vi "Unregister.vi"(8 "Error In":errorcluster, 10 "Registrant Enq":refnum<class "Message Enqueuer.lvclass">, 11 "Event Source In":refnum<class "Event Source Actor.lvclass">) -> (0 "Error Out":errorcluster, 3 "Event Source Out":refnum<class "Event Source Actor.lvclass">)   [LabVIEW 2021, in "EventSourceActor.lvlib" / "Event Source.lvlib" / "Event Source Actor.lvclass"]
doc: "This method unregisters a specific Actors Enqueuer from all Events he is listening to from this Event Source Actor."
uses:
  Event Source Actor.lvclass
  <vilib>/ActorFramework/Message Enqueuer/Message Enqueuer.lvclass
  Event Source Actor.lvclass/Event Source Actor.ctl
  48172011-38dd-4e95-b88c-c50fd512a03c.vi
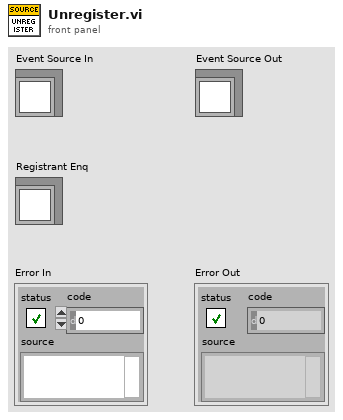
[diagram p1: front panel]
types:
  T1 = map{string, set{refnum<class "Message Enqueuer.lvclass">}}
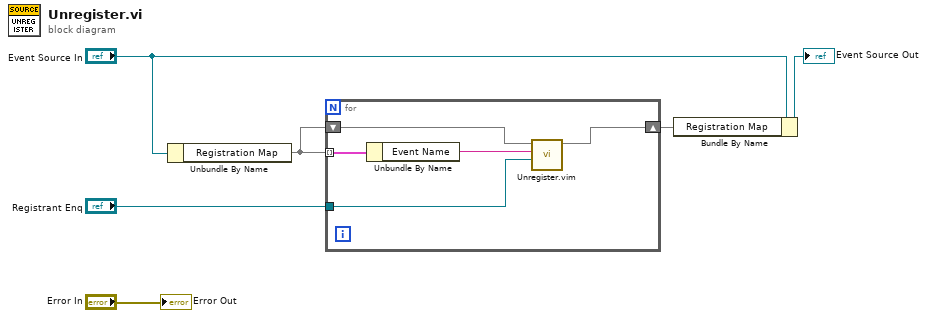
[diagram p0: block diagram]
diagram:
  n1 = Unbundle By Name("Event Source In") -> ("Registration Map"=w6:T1)
  n2 = for {
    tunnel: w6 -> [w11] mode=indexing
    shift-right: [w7] -> w4
    shift-left: w6 -> [w9]
    tunnel: "Registrant Enq" -> [w8]
    n3 = Unbundle By Name(w11) -> ("Event Name"=w10:string)
    n4 = call "Unregister.vim"("set element"=w8, "key"=w10, "map in"=w9) -> ("map out"=w7:T1)  [unwired: 6 in, 2 out]
  }
  n5 = Bundle By Name(cluster="Event Source In", "Registration Map"=w4) -> (→"Event Source Out":refnum<class "Event Source Actor.lvclass">)
  "Error Out" <- "Error In"
